vi "Localize_Particles_without_LoG-1.vi"(4 "# channel":u8, 5 "[IN] Filtering settings":T1, 6 "[IN] Destination Image":T2, 7 "error IN":errorcluster, 10 "[IN] Frame":T2) -> (0 "error OUT":errorcluster, 2 "Histogram Graph":T3 {"Incremental Value" format="%.2f"; "Starting Value" format="%.2f"}, 3 "[OUT] Processed Image":T2)   [LabVIEW 2013]
uses:
  <vilib>/vision/Image Controls.llb/IMAQ Image.ctl
  <vilib>/vision/NI_Vision_Development_Module.lvlib
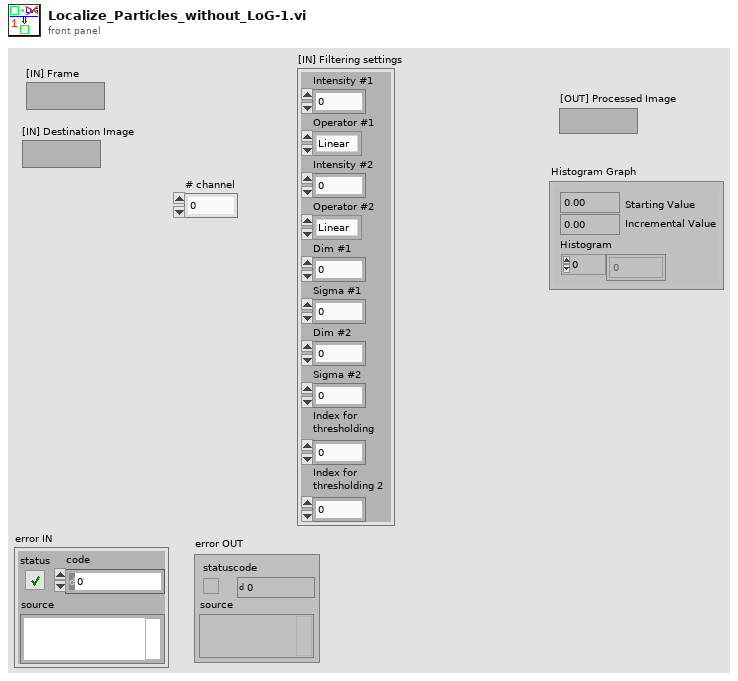
[diagram p1: front panel]
types:
  T1 = cluster{"Intensity #1":sgl, "Operator #1":enum32{"Linear", "Log", "Exp", "Square", "Square root", "Power X", "Power 1/X"}, "Intensity #2":sgl, "Operator #2":enum32{"Linear", "Log", "Exp", "Square", "Square root", "Power X", "Power 1/X"}, "Dim #1":u8, "Sigma #1":dbl, "Dim #2":u8, "Sigma #2":dbl, "Index for \nthresholding":i8, "Index for \nthresholding 2":i8}
  T2 = typedef "IMAQ Image.ctl" = refnum<image>
  T3 = cluster{"Starting Value":sgl, "Incremental Value":sgl, "Histogram":u32[]}
  T4 = enum32{"Linear", "Log", "Exp", "Square", "Square root", "Power X", "Power 1/X"}
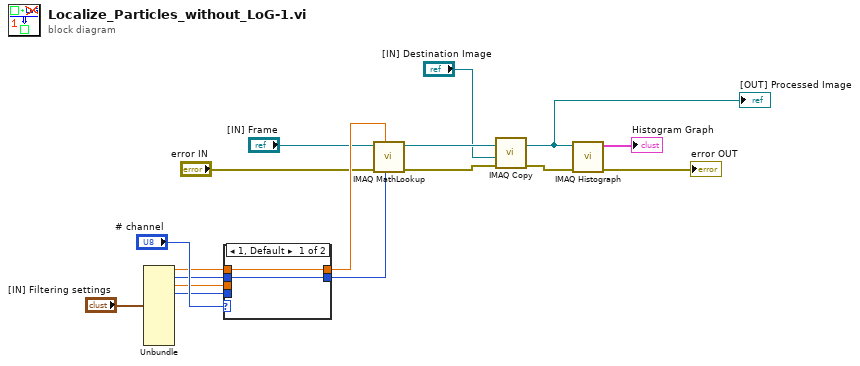
[diagram p0: block diagram]
diagram:
  n1 = Unbundle("[IN] Filtering settings") -> ("Intensity #1"=w14:sgl, "Operator #1"=w13:T4, "Intensity #2"=w10:sgl, "Operator #2"=w9:T4)  [unwired: 6 out]
  n2 = case shown="1, Default" "# channel" {
    tunnel: w14 -> [w19 _]
    tunnel: w13 -> [w18 _]
    tunnel: [w19 w21] -> w12
    tunnel: [w18 w20] -> w11
    tunnel: w10 -> [_ w21]
    tunnel: w9 -> [_ w20]
    frame 1, Default {
    }
    frame 2 {
    }
  }
  n3 = call "IMAQ MathLookup"("Operator"=w11, "X Value"=w12, "error in (no error)"="error IN", "Image Src"="[IN] Frame") -> ("error out"=w3:errorcluster, "Image Dst Out"=w5:T2)  [unwired: 6 in]
  n4 = call "IMAQ Copy"("error in (no error)"=w3, "Image Dst"="[IN] Destination Image", "Image Src"=w5) -> ("error out"=w1:errorcluster, "Image Dst Out"=w2:T2)  [unwired: 3 in]
  "[OUT] Processed Image" <- w2
  n5 = call "IMAQ Histograph"("error in (no error)"=w1, "Image"=w2) -> ("error out"=→"error OUT":errorcluster, "Histogram Graph"=→"Histogram Graph":T3)  [unwired: 6 in, 2 out]
